vi "test-buttonColumn.vi"(8 "error in (no error)":errorcluster, 10 "ColumnSetup":T1[](array[typedef]) {"MinWidth" min=2 step=1; "AutoSizeMode" items=["None"=1, "ColumnHeader"=2, "AllCellsExceptHeader"=4, "AllCells"=6, "DisplayedCellsExceptHeader"=8, "DisplayedCells"=10, "Fill"=16]; "FillWeight" min=1 max=100}, 11 ".NET Refnum in":refnum<k24>) -> (0 "error out":errorcluster)   [LabVIEW 2014]
uses:
  System.Windows.Forms
  GridColumn/ColumnDefinition.ctl
  GridColumn/GridColumn.lvclass
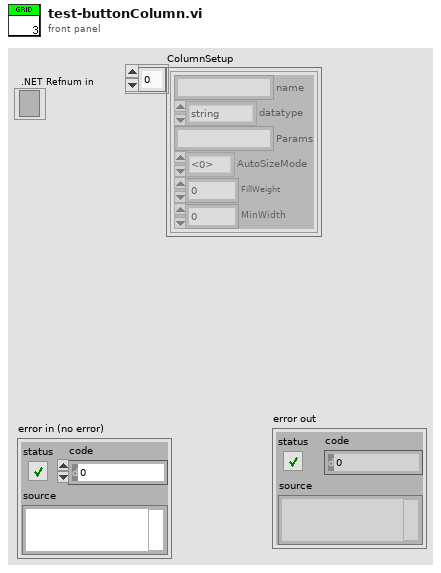
[diagram p1: front panel]
types:
  T1 = typedef "GridColumn.lvclass/ColumnDefinition.ctl" = cluster{"name":string, "datatype":enum16{"string", "image", "check", "numeric", "timestamp", "button", "combo"}, "Params":string, "AutoSizeMode":i32, "FillWeight":sgl, "MinWidth":i32}
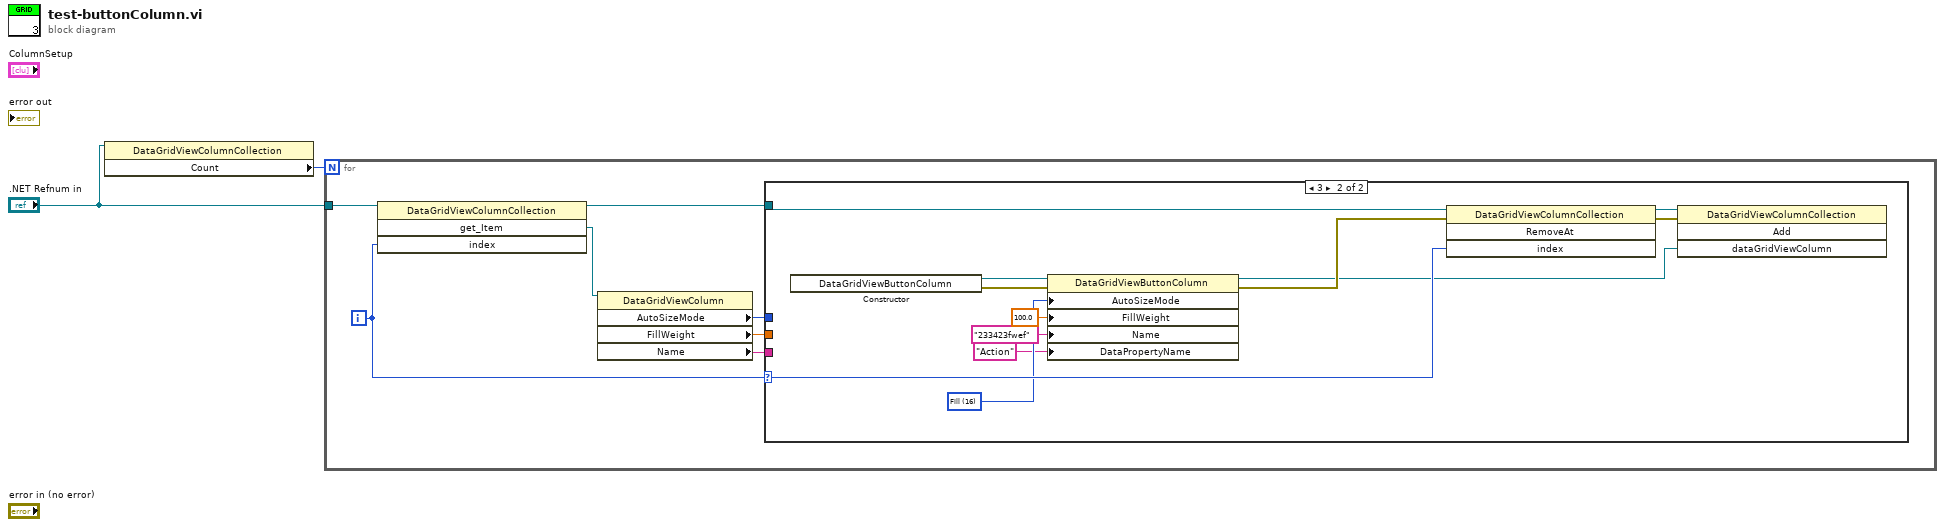
[diagram p0: block diagram]
diagram:
  n1 = property class="DataGridViewColumnCollection"(reference=".NET Refnum in") -> ("Count"=w1:i32)  [unwired: 1 in, 2 out]
  n2 = for {
    N: w1 -> [_]
    tunnel: ".NET Refnum in" -> [w9]
    i -> [w7]
    n3 = invoke class="DataGridViewColumnCollection" method="get_Item"(reference=w9, "index"=w7) -> (reference out=w6:refnum<k24>, "get_Item"=w8:refnum<k24>)  [unwired: 2 in, 2 out]
    n4 = property class="DataGridViewColumn"(reference=w8) -> ("AutoSizeMode"=w5:i32, "FillWeight"=w4:sgl, "Name"=w3:string)  [unwired: 1 in, 2 out]
    n5 = case shown="3" w7 {
      selector: w7 -> [_ w20]
      tunnel: w6 -> [_ w21]
      tunnel: w5 -> [_ _]
      tunnel: w4 -> [_ _]
      tunnel: w3 -> [_ _]
      frame Default {
      }
      frame 3 {
        w13 = 16 items=["NotSet"=0, "None"=1, "ColumnHeader"=2, "AllCellsExceptHeader"=4, "AllCells"=6, "DisplayedCellsExceptHeader"=8, "DisplayedCells"=10, "Fill"=16] ("AutoSizeMode")
        n6 = constructor class="DataGridViewButtonColumn"() -> (reference out=w17:refnum<k24>, error out=w16:errorcluster)  [unwired: 3 in, 1 out]
        n7 = property class="DataGridViewButtonColumn"(reference=w17, error in=w16, "AutoSizeMode"=w13, "FillWeight"=sgl 100.0, "Name"="233423fwef", "DataPropertyName"="Action") -> (reference out=w14:refnum<k24>, error out=w15:errorcluster)
        n8 = invoke class="DataGridViewColumnCollection" method="RemoveAt"(reference=w21, error in=w15, "index"=w20) -> (reference out=w19:refnum<k24>, error out=w18:errorcluster)  [unwired: 1 in, 2 out]
        n9 = invoke class="DataGridViewColumnCollection" method="Add"(reference=w19, error in=w18, "dataGridViewColumn"=w14) -> ()  [unwired: 1 in, 4 out]
      }
    }
  }
